vi "fontmontant detector.vi"   [LabVIEW 2019]
uses:
  <vilib>/eio/EIONode/EIONode.xnode
  <vilib>/rvi/eio/common/nirviEmuTemplateMethod_errors.vi
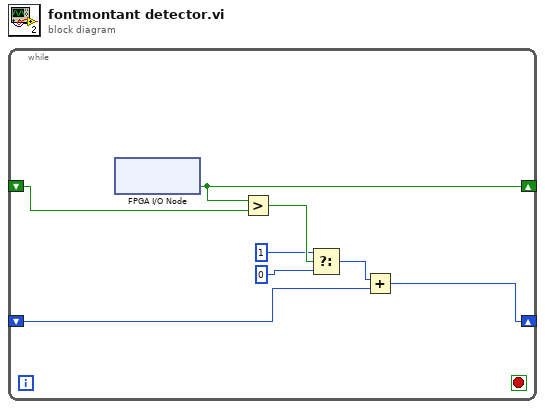
[diagram p0: block diagram]
diagram:
  n1 = while {
    shift-right: [w8] -> _
    shift-left: _ -> [w7]
    shift-right: [w1] -> _
    shift-left: _ -> [w3]
    stop <- _ stop-if-true
    n2 = xnode "FPGA I/O Node"() -> ("Button0"=w8:bool)  [unwired: 1 in, 1 out]
    n3 = Greater?(x=w8, y=w7) -> (0:w6:bool)
    n4 = Select(t=i16 1, s=w6, f=i16 0) -> (s? t:f=w2:i16)
    n5 = Add(x=w2, y=w3) -> (x+y=w1:i16)
  }
